vi "Output FGV.vi"(4 "error in":errorcluster, 6 "Function":enum16{"write", "read"}(ring), 7 "Output":waveform(dbl)[][](array[waveform])=[[{"t0"=timestamp(0 s since 1904-01-01), "dt"=5.17729651930355e-06, "Y"=array[14350 elements]}, {"t0"=timestamp(0 s since 1904-01-01), "dt"=5.17729651930355e-06, "Y"=array[14350 elements]}], [{"t0"=timestamp(0 s since 1904-01-01), "dt"=5.17729651930355e-06, "Y"=array[14350 elements]}, {"t0"=timestamp(0 s since 1904-01-01), "dt"=5.17729651930355e-06, "Y"=array[14350 elements]}], [{"t0"=timestamp(0 s since 1904-01-01), "dt"=5.17729651930355e-06, "Y"=array[14350 elements]}, {"t0"=timestamp(0 s since 1904-01-01), "dt"=5.17729651930355e-06, "Y"=array[14350 elements]}], [{"t0"=timestamp(0 s since 1904-01-01), "dt"=5.17729651930355e-06, "Y"=array[14350 elements]}, {"t0"=timestamp(0 s since 1904-01-01), "dt"=5.17729651930355e-06, "Y"=array[14350 elements]}]]) -> (0 "error out":errorcluster, 3 "Output":waveform(dbl)[][](array[waveform])=[[{"t0"=timestamp(0 s since 1904-01-01), "dt"=5.17729651930355e-06, "Y"=array[14350 elements]}, {"t0"=timestamp(0 s since 1904-01-01), "dt"=5.17729651930355e-06, "Y"=array[14350 elements]}], [{"t0"=timestamp(0 s since 1904-01-01), "dt"=5.17729651930355e-06, "Y"=array[14350 elements]}, {"t0"=timestamp(0 s since 1904-01-01), "dt"=5.17729651930355e-06, "Y"=array[14350 elements]}], [{"t0"=timestamp(0 s since 1904-01-01), "dt"=5.17729651930355e-06, "Y"=array[14350 elements]}, {"t0"=timestamp(0 s since 1904-01-01), "dt"=5.17729651930355e-06, "Y"=array[14350 elements]}], [{"t0"=timestamp(0 s since 1904-01-01), "dt"=5.17729651930355e-06, "Y"=array[14350 elements]}, {"t0"=timestamp(0 s since 1904-01-01), "dt"=5.17729651930355e-06, "Y"=array[14350 elements]}]])   [LabVIEW 2013]
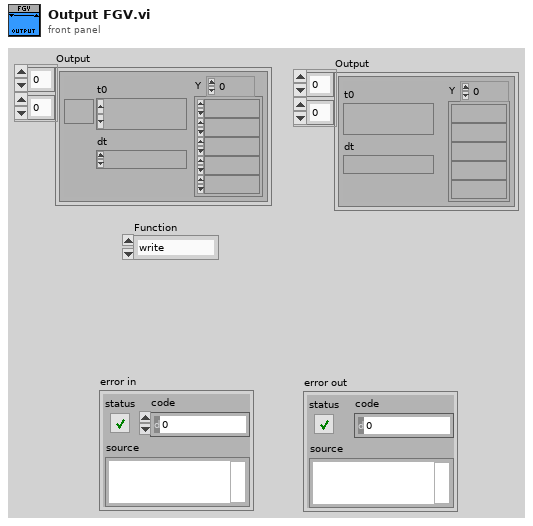
[diagram p1: front panel]
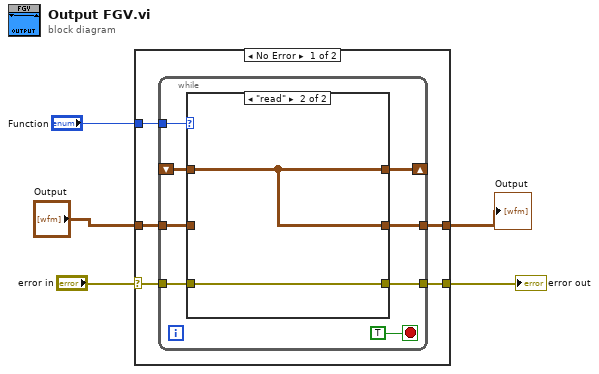
[diagram p0: block diagram]
diagram:
  n1 = case shown="No Error" "error in" {
    selector: "error in" -> [w10 w24]
    tunnel: [w9 w24] -> w4
    tunnel: "Output" -> [w8 w23]
    tunnel: [w7 w23] -> w1
    tunnel: "Function" -> [w6 _]
    frame No Error {
      n2 = while {
        shift-right: [w12] -> _
        shift-left: _ -> [w11]
        tunnel: w10 -> [w17]
        tunnel: [w16] -> w9
        tunnel: w8 -> [w15]
        tunnel: [w14] -> w7
        tunnel: w6 -> [w13]
        stop <- TRUE stop-if-true
        n3 = case shown="\"read\"" w13 {
          tunnel: w17 -> [w19 w22]
          tunnel: [w19 w22] -> w16
          tunnel: w15 -> [w20 _]
          tunnel: [w20 w21] -> w14
          tunnel: [w20 w21] -> w12
          tunnel: w11 -> [_ w21]
          frame "write", Default {
          }
          frame "read" {
          }
        }
      }
    }
    frame Error {
    }
  }
  "error out" <- w4
  "Output" <- w1
